vi "microflow_mass_flow.vi"(1 "Source Offset":dbl format="%#_13g", 2 "Source":dbl[](array[numeric]) format="%#_13g", 3 "Target Low":dbl format="%#_13g", 4 "Target High":dbl=377.9933 format="%#_13g") -> (0 "Target":dbl[](array[numeric]) format="%#_13g")   [LabVIEW 2017, in "sensor_translation.lvlib"]
uses:
  sensor_translation.lvlib
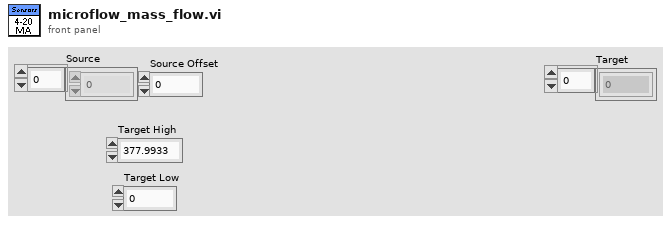
[diagram p1: front panel]
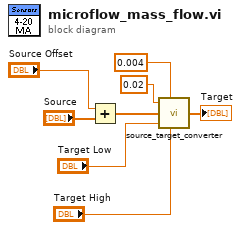
[diagram p0: block diagram]
diagram:
  n1 = Add(x="Source Offset", y="Source") -> (x+y=w1:dbl[])
  n2 = call "source_target_converter.vi"("Source High"=0.02, "Source Low"=0.004, "Source"=w1, "Target Low"="Target Low", "Target High"="Target High") -> ("Target"=→"Target":dbl[])
